vi "OAT Envelope Detection (Even Angle Output, N Channels).vi"(0 "scaled signals [EU]":waveform(dbl)[](array[waveform]), 1 "reset? (F)":bool, 5 "speed profile":T6 {"speed [RPM]" format="%.2f"; "time [s]" format="%.2f"}, 7 "pulse/revolution (1)":i32=1, 9 "band specification":T1, 11 "error in (no error)":errorcluster) -> (4 "even-angle envelope signals":cluster{"r0":dbl, "dr":dbl, "Y":dbl[]}[](array[cluster]) {"r0" format="%.2p"; "dr" format="%.2p"; "Y" format="%.2f"}, 6 "even-angle channel info":T2[](array[typedef]) {"channel info"."pregain" format="%.2f"; "channel info"."weighting filter" items=["Linear", "A-weighting", "B-weighting", "C-weighting", "ITU-R 468-4", "Dolby", "CCITT", "C-message", "Wb", "Wc", "Wd", "We", "Wf", "Wh", "Wj", "Wk", "Wm", "AES17 20 kHz lowpass", "AES17 40 kHz lowpass", "AES17 20 kHz highpass", "AES17 40 kHz highpass"]; "channel info"."dB reference" format="%^.1e"; "channel info"."engineering units" items=["custom..."=0, "V"=1, "A"=21, "C"=30, "pC"=31, "s"=32, "-"=29, "Pa"=2, "N"=20, "g"=3, "m/s^2"=4, "m/s"=5, "m"=6, "mm/s"=12, "mm"=13, "micron/s"=14, "micron"=15, "in/s^2"=7, "in/s"=8, "in"=9, "mil/s"=10, "mil"=11, "rad/s^2"=16, "rad/s"=17, "rad"=18, "deg/s^2"=26, "deg/s"=27, "deg"=28, "RPM"=22, "cycle/s^2"=23, "Hz"=24, "cycle"=25, "strain"=19]; "channel info"."sensor sensitivity" format="%#_5f"}, 14 "actual max order":dbl, 15 "error out":errorcluster)   [LabVIEW 2017, in "SoundVib_FaultAnalysis.lvlib"]
doc: "Extracts the modulating signal, or envelope signal, from an amplitude-modulated signal. You can use the envelope detection technique to identify the mechanical faults that have amplitude-modulating effect on the vibration signal of a machine. Wire data to the <B>scaled signal [EU]</B> input to determine the polymorphic instance to use or manually select the instance."
uses:
  <vilib>/addons/Sound and Vibration/Order Analysis/Fault Analysis/SoundVib_FaultAnalysis.lvlib
  <vilib>/addons/Sound and Vibration/Order Analysis/Tach Process/SubVIs/speed profile.ctl
  <vilib>/addons/_NISVFA/_Shared subVIs/Controls/svc_Resampled Channel Info.ctl
  <vilib>/addons/_NISVFA/_Shared subVIs/Controls/svc_Channel Info.ctl
  <vilib>/addons/_NISVFA/_Shared subVIs/Controls/svc_Engineering Units Text Ring.ctl
  <vilib>/addons/_NISVFA/_Shared subVIs/Controls/svc_Weighting Filter Text Ring.ctl
  <vilib>/addons/_NISVFA/_Shared subVIs/Common/svc_Check for Waveform Parameter Continuity (no state).vi
  <vilib>/addons/Sound and Vibration/Order Analysis/Resample Order Tracking/SubVIs/oa_Calculate CIC Decimation Filter Coefficients.vi
  <vilib>/addons/Sound and Vibration/Order Analysis/Fault Analysis/SubVIs/sv_Compute Shift and Low Pass Filter with IC.vi
  <vilib>/addons/_NISVFA/_Shared subVIs/Common/svc_Get SV Channel Info.vi
  <vilib>/addons/Sound and Vibration/Order Analysis/Resample Order Tracking/SubVIs/oa_Decimation with CIC and Compensation Filter.vi
  <vilib>/addons/Sound and Vibration/Order Analysis/Fault Analysis/SubVIs/oa_Demodulation Initial States (1 Channel).vi
  <vilib>/addons/Sound and Vibration/Order Analysis/Adv Resampling/OAT Single Stage Decimation with IC.vi
  <vilib>/addons/Sound and Vibration/Order Analysis/Resample Order Tracking/SubVIs/OAT CIC Decimation.vi
  <vilib>/addons/Sound and Vibration/Order Analysis/Resample Order Tracking/SubVIs/oa_Interpolate Zeros Between Samples.vi
  <vilib>/addons/Sound and Vibration/Order Analysis/Resample Order Tracking/SubVIs/oa_Calculate Delay of CIC Decimation Interpolation Filter.vi
  <vilib>/addons/Sound and Vibration/Order Analysis/Resample Order Tracking/SubVIs/oa_Create CIC Compensation Filter.vi
  <vilib>/addons/Sound and Vibration/Order Analysis/Resample Order Tracking/SubVIs/oa_Create CIC LP Truncation Filter.vi
  <vilib>/addons/Sound and Vibration/Order Analysis/Resample Order Tracking/OAT Convert to Even Angle Signal (N Channels).vi
  <vilib>/addons/_NISVFA/_Shared subVIs/Common/svc_Engineering Units to Unit Label.vi
  <vilib>/addons/_NISVFA/_Shared subVIs/Common/svc_Unit Label to Engineering Units.vi
  <vilib>/addons/Sound and Vibration/Order Analysis/Resample Order Tracking/SoundVib_Resampling.lvlib
  <vilib>/addons/Sound and Vibration/Order Analysis/Resample Order Tracking/SoundVib_OrderTracking.lvlib
  <vilib>/Analysis/NI_AALPro.lvlib
  <vilib>/addons/Sound and Vibration/Order Analysis/Tach Process/SoundVib_TachProcess.lvlib
panel:
  in  "empty waveform":waveform(dbl)[](array[waveform])
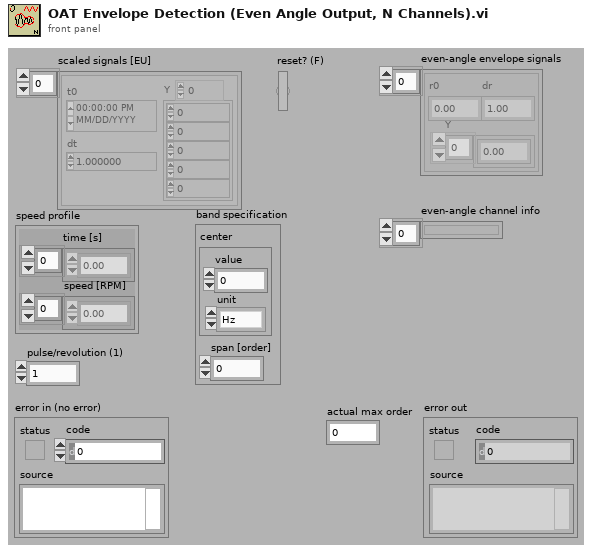
[diagram p1: front panel]
types:
  T1 = cluster{"center":cluster{"value":dbl, "unit":enum16{"Hz", "order"}}, "span [order]":dbl}
  T2 = typedef "svc_Resampled Channel Info.ctl" = cluster{"channel name":string, "description":string, " channel info":T3}
  T3 = typedef "svc_Channel Info.ctl" = cluster{"sensor sensitivity":dbl, "engineering units":T4, "dB reference":dbl, "custom label":string, "weighting filter":T5, "pregain":dbl}
  T4 = typedef "svc_Engineering Units Text Ring.ctl" = u16
  T5 = typedef "svc_Weighting Filter Text Ring.ctl" = u16
  T6 = typedef "SoundVib_TachProcess.lvlib/speed profile.ctl" = cluster{"time [s]":dbl[], "speed [RPM]":dbl[]}
  T7 = cluster{"dt equal":bool, "array length equal":bool, "number channels change":bool}
  T8 = cluster{"dt":bool, "t0 continuity":bool, "array length":bool, "channel info":bool, "name":bool}
  T9 = typedef "OAT Decimation Filter.ctl" = cluster{"coefficients":dbl[], "factor":i32}
  T10 = cluster{"filter settings":cluster{"CIC Settings":cluster{"Numeric":i32, i32, i32}, "filters":T9[], "delay":i32, "interpolation factor":i32}, "filter states":cluster{"t0":dbl, "phase":dbl, "real filter state":cluster{cluster{dbl[]}, cluster{dbl[]}[]}, "imaginary filter state":cluster{cluster{dbl[]}, cluster{dbl[]}[]}, "delay":i32}[], "reset pending":bool}
  T11 = cluster{"t0 out":dbl, "new dt":dbl, "enveloped signals":dbl[]}
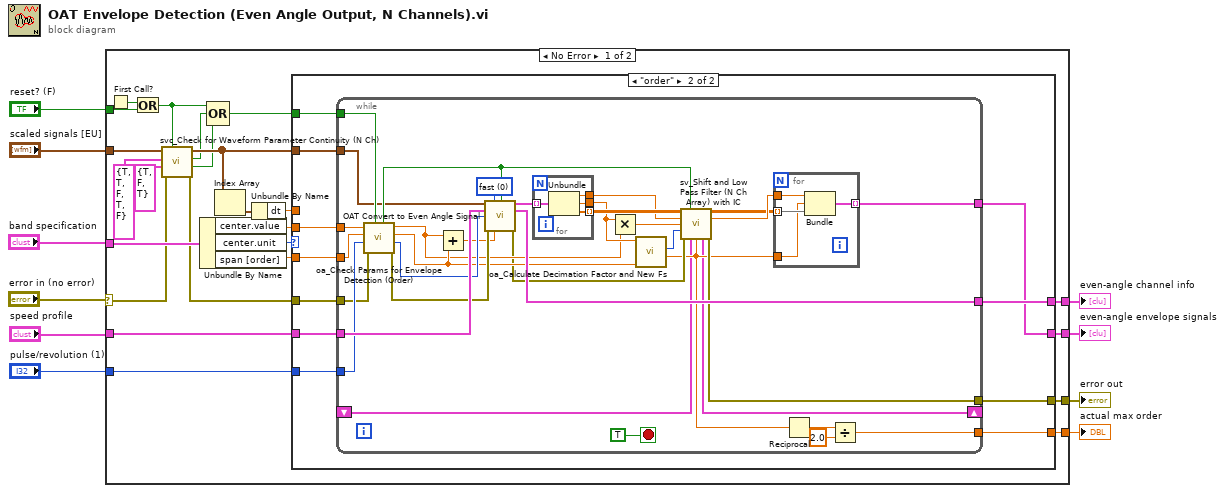
[diagram p0: block diagram]
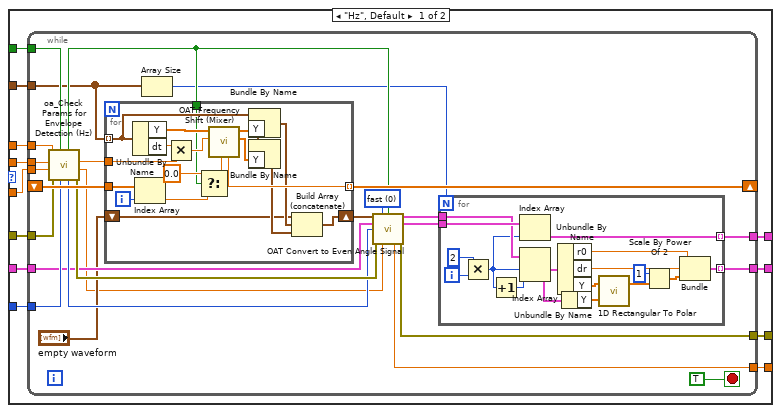
[diagram p2: hidden frame]
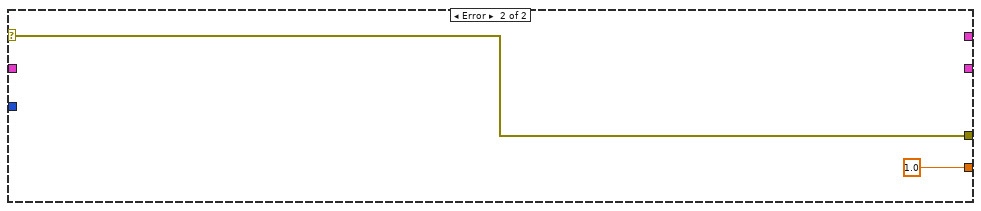
[diagram p3: hidden frame]
diagram:
  n1 = case shown="No Error" "error in (no error)" {
    selector: "error in (no error)" -> [w18 w161]
    tunnel: [w32 w161] -> w2
    tunnel: "speed profile" -> [w34 _]
    tunnel: "pulse/revolution (1)" -> [w27 _]
    tunnel: [w33 _] -> w4
    tunnel: [w31 _] -> w3
    tunnel: "reset? (F)" -> [w29 _]
    tunnel: "band specification" -> [w26 _]
    tunnel: "scaled signals [EU]" -> [w23 _]
    tunnel: [w20 1.0 ("actual max order")] -> w1
    frame No Error {
      n2 = First Call?() -> (First Call?: T/F=w30:bool)
      n3 = Or(x=w30, y=w29) -> (x .or. y?=w13:bool)
      n4 = call <vilib>:"svc_Check for Waveform Parameter Continuity (N Ch).vi"("restart averaging (F)"=w13, "error in (no error)"=w18, "checks for multichannel parameters"=T7 {"dt equal"=TRUE, "array length equal"=FALSE, "number channels change"=TRUE}, "checks for channel parameter change"=T8 {"dt"=TRUE, "t0 continuity"=TRUE, "array length"=FALSE, "channel info"=TRUE, "name"=FALSE}, "scaled signal(s)"=w23) -> ("error out"=w17:errorcluster, "multichannel parameter changed"=w14:bool, "waveform parameter changed"=w15:bool, "dup scaled signal(s)"=w19:waveform(dbl)[])  [unwired: 3 out]
      n5 = Unbundle By Name(w26) -> ("center.value"=w25:dbl, "center.unit"=w28:enum16{"Hz", "order"}, "span [order]"=w24:dbl)
      n6 = Compound Arithmetic op=OR(w13, w15, w14) -> (w16:bool)
      n7 = Index Array(array=w19) -> (element=w22:waveform(dbl))  [unwired: 1 in]
      n8 = Unbundle By Name(w22) -> ("dt"=w21:dbl)
      n9 = case shown="\"order\"" w28 {
        tunnel: w19 -> [w46 w118]
        tunnel: w34 -> [w45 w117]
        tunnel: [w39 w116] -> w33
        tunnel: w17 -> [w44 w115]
        tunnel: [w38 w114] -> w32
        tunnel: [w37 w109] -> w31
        tunnel: w16 -> [w43 w113]
        tunnel: w27 -> [w42 w112]
        tunnel: w25 -> [w41 w110]
        tunnel: w24 -> [w40 w111]
        tunnel: w21 -> [w36 _]
        tunnel: [w35 w108] -> w20
        frame "Hz", Default {
          n10 = while {
            tunnel: w43 -> [w67]
            tunnel: w46 -> [w50]
            tunnel: w45 -> [w59]
            tunnel: w42 -> [w68]
            tunnel: w44 -> [w69]
            shift-right: [w71] -> _
            shift-left: _ -> [w72]
            tunnel: w41 -> [w66]
            tunnel: w40 -> [w65]
            tunnel: [w56] -> w39
            tunnel: [w55] -> w38
            tunnel: [w54] -> w37
            tunnel: w36 -> [w48]
            tunnel: [w47] -> w35
            stop <- TRUE stop-if-true
            w63 = u16 0 items=["fast", "accurate"] ("analysis method")
            n11 = call <vilib>:"oa_Check Params for Envelope Detection (Hz).vi"("pulse/revolution (1)"=w68, "reset"=w67, "error in (no error)"=w69, "span"=w65, "center"=w66, "dt"=w48) -> ("error out"=w61:errorcluster, "span out"=w52:dbl, "center out"=w64:dbl, "pulse/revolution out"=w60:i32, "reset out"=w51:bool)  [unwired: 1 out]
            n12 = for {
              tunnel: w72 -> [w96]
              tunnel: [w102] -> w71 mode=indexing
              tunnel: w51 -> [w93]
              tunnel: w50 -> [w94] mode=indexing
              tunnel: w64 -> [w92]
              shift-right: [w91] -> w62
              shift-left: "empty waveform" -> [w90]
              i -> [w95]
              n13 = Unbundle By Name(w94) -> ("Y"=w107:dbl[], "dt"=w106:dbl)
              n14 = Index Array(array=w96, index=w95) -> (element=w97:dbl)
              n15 = Multiply(x=w106, y=w92) -> (x*y=w105:dbl)
              n16 = Select(t=0.0, s=w93, f=w97) -> (s? t:f=w103:dbl)
              n17 = call <vilib>:"OAT Frequency Shift (Mixer).vi"("initial phase"=w103, "fc"=w105, "X"=w107) -> ("imaginary"=w100:dbl[], "real"=w101:dbl[], "final phase"=w102:dbl)  [unwired: 6 in]
              n18 = Bundle By Name(cluster=w94, "Y"=w101) -> (w99:waveform(dbl))
              n19 = Bundle By Name(cluster=w94, "Y"=w100) -> (w98:waveform(dbl))
              n20 = Build Array (concatenate)(w90, w99, w98) -> (w91:waveform(dbl)[])
            }
            n21 = Array Size(array=w50) -> (size(s)=w49:i32)
            n22 = call-poly <vilib>:"OAT Convert to Even Angle Signal.vi"("scaled signals [EU]"=w62, "analysis method"=w63, "reset? (F)"=w51, "speed profile"=w59, "pulse/revolution (1)"=w60, "error in (no error)"=w61, "max order (auto)"=w52) -> ("even-angle signals"=w57:cluster{"r0":dbl, "dr":dbl, "Y":dbl[]}[], "even-angle channel info"=w58:T2[], "actual max order"=w47:dbl, "error out"=w55:errorcluster)  [unwired: 4 in, 1 out]
            n23 = for {
              N: w49 -> [_]
              tunnel: w58 -> [w87]
              tunnel: w57 -> [w84]
              tunnel: [w83] -> w56 mode=indexing
              tunnel: [w76] -> w54 mode=indexing
              i -> [w86]
              n24 = Multiply(x=2, y=w86) -> (x*y=w80:i32)
              n25 = Increment(x=w80) -> (x+1=w79:i32)
              n26 = Index Array(array=w87, index=w80) -> (element=w83:T2)
              n27 = Index Array(array=w84, index #1=w80, index #2=w79) -> (element #1=w82:cluster{"r0":dbl, "dr":dbl, "Y":dbl[]}, element #2=w81:cluster{"r0":dbl, "dr":dbl, "Y":dbl[]})
              n28 = Unbundle By Name(w82) -> ("r0"=w88:dbl, "dr"=w89:dbl, "Y"=w78:dbl[])
              n29 = Unbundle By Name(w81) -> ("Y"=w77:dbl[])
              n30 = call <vilib>:"1D Rectangular To Polar.vi"("X"=w78, "Y"=w77) -> ("Magnitude"=w74:dbl[])  [unwired: 2 out]
              n31 = Scale By Power Of 2(n=1, x=w74) -> (x*2^n=w75:dbl[])
              n32 = Bundle("r0"=w88, "dr"=w89, w75) -> (w76:cluster{"r0":dbl, "dr":dbl, dbl[]})  [unwired: 1 in]
            }
          }
        }
        frame "order" {
          n33 = while {
            tunnel: w113 -> [w148]
            tunnel: w118 -> [w140]
            tunnel: w117 -> [w151]
            tunnel: w112 -> [w147]
            tunnel: [w142] -> w116
            tunnel: w115 -> [w145]
            tunnel: [w126] -> w114
            tunnel: w111 -> [w139]
            tunnel: w110 -> [w138]
            tunnel: [w132] -> w109
            tunnel: [w122] -> w108
            shift-right: [w120] -> _
            shift-left: _ -> [w119]
            stop <- TRUE stop-if-true
            w150 = u16 0 items=["fast", "accurate"] ("analysis method")
            n34 = call <vilib>:"oa_Check Params for Envelope Detection (Order).vi"("reset"=w148, "error in (no error)"=w145, "pulse/revolution (1)"=w147, "span [Order]"=w139, "center"=w138) -> ("error out"=w144:errorcluster, "pulse/revolution out"=w146:i32, "span [Order] out"=w137:dbl, "center out"=w128:dbl, "reset out"=w141:bool)  [unwired: 2 in]
            n35 = Add(x=w128, y=w137) -> (x+y=w143:dbl)
            n36 = call-poly <vilib>:"OAT Convert to Even Angle Signal.vi"("scaled signals [EU]"=w140, "analysis method"=w150, "reset? (F)"=w141, "speed profile"=w151, "pulse/revolution (1)"=w146, "error in (no error)"=w144, "max order (auto)"=w143) -> ("even-angle signals"=w135:cluster{"r0":dbl, "dr":dbl, "Y":dbl[]}[], "even-angle channel info"=w142:T2[], "error out"=w127:errorcluster)  [unwired: 4 in, 2 out]
            n37 = for {
              tunnel: w135 -> [w159] mode=indexing
              tunnel: [w158] -> w134 mode=indexing
              tunnel: [w157] -> w133
              tunnel: [w156] -> w129
              n38 = Unbundle(w159) -> ("r0"=w157:dbl, "dr"=w156:dbl, "Y"=w158:dbl[])
            }
            n39 = Multiply(x=w129, y=w128) -> (x*y=w130:dbl)
            n40 = call <vilib>:"oa_Calculate Decimation Factor and New Fs.vi"("span"=w137, "dt"=w129) -> ("new dt"=w125:dbl, "decimation factor"=w136:i32)  [unwired: 8 in]
            n41 = call <vilib>:"sv_Shift and Low Pass Filter (N Ch Array) with IC.vi"("input signals"=w134, "reset? (F)"=w141, "t0"=w133, "center"=w130, "decimation factor"=w136, "error in (no error)"=w127, "initial conditions"=w119, "new dt"=w125) -> ("enveloped signals"=w121:dbl[][], "t0 out"=w131:dbl, "final conditions"=w120:T10, "error out"=w126:errorcluster)  [unwired: 4 in]
            n42 = for {
              tunnel: w121 -> [w155] mode=indexing
              tunnel: w125 -> [w154]
              tunnel: w131 -> [w153]
              tunnel: [w152] -> w132 mode=indexing
              n43 = Bundle("t0 out"=w153, "new dt"=w154, "enveloped signals"=w155) -> (w152:T11)  [unwired: 1 in]
            }
            n44 = Reciprocal(x=w125) -> (1/x=w124:dbl)
            n45 = Divide(x=w124, y=2.0) -> (x/y=w122:dbl)
          }
        }
      }
    }
    frame Error {
    }
  }
  "error out" <- w2
  "even-angle envelope signals" <- w3
  "even-angle channel info" <- w4
  "actual max order" <- w1
